vi "cDAQ DDS Open.vi"(8 "error in":errorcluster, 11 "session in":T1={"device"="", "channels"=[], "mclk source"="", "mclk [Hz]"=0.0, "fs [Hz]"=0.0, "block [s]"=0.0, "buf [s]"=0.0, "task"="", "cmd queue"=refnum, "proc ref"=refnum, "smpl clock out"="/cDAQ3/PFI0", "export smpl clock"=FALSE, "DC ofs [V]"=[], "timebase source"="", "timebase mode"=enum."Local"} {"channels" min=0 step=1}) -> (0 "error out":errorcluster, 2 "idn string":string, 3 "session out":T1={"device"="", "channels"=[], "mclk source"="", "mclk [Hz]"=0.0, "fs [Hz]"=0.0, "block [s]"=0.0, "buf [s]"=0.0, "task"="", "cmd queue"=refnum, "proc ref"=refnum, "smpl clock out"="/cDAQ3/PFI0", "export smpl clock"=FALSE, "DC ofs [V]"=[], "timebase source"="", "timebase mode"=enum."Local"} {"channels" min=0 step=1})   [LabVIEW 2020]
uses:
  cDAQ DDS Session.ctl
  cDAQ DDS Setup.ctl
  cDAQ DDS Timebase Mode.ctl
  <vilib>/Utility/error.llb/Error Cluster From Error Code.vi
  <vilib>/DAQmx/create/channels.llb/DAQmx Create Channel (AO-Voltage-Basic).vi
  <vilib>/ErrorRing/Error Ring.xnode
  <resource>/objmgr/daqmx.rc
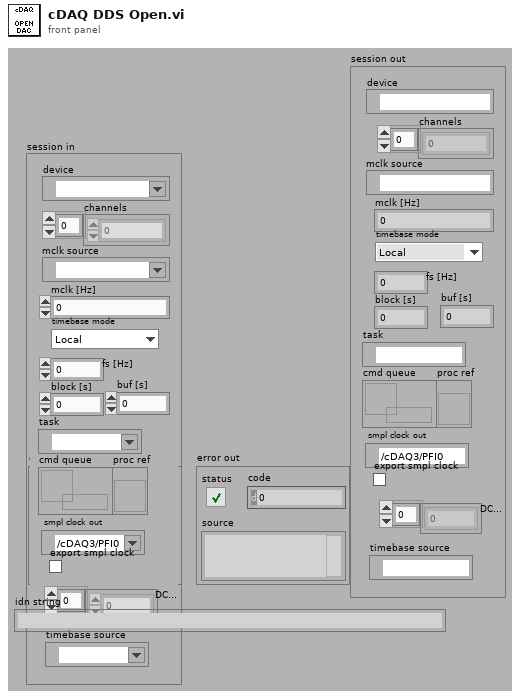
[diagram p1: front panel]
types:
  T1 = typedef "cDAQ DDS Session.ctl" = cluster{"device":tag, "channels":i32[], "mclk source":tag, "mclk [Hz]":dbl, "fs [Hz]":dbl, "block [s]":dbl, "buf [s]":dbl, "task":refnum<k21>, "cmd queue":refnum<queue>, "proc ref":refnum<vi>, "smpl clock out":tag, "export smpl clock":bool, "DC ofs [V]":dbl[], "timebase source":tag, "timebase mode":T2}
  T2 = typedef "cDAQ DDS Timebase Mode.ctl" = enum16{"Local", "Take from ADC (e.g. NI 9238)", "Other source"}
  T3 = typedef "cDAQ DDS Setup.ctl" = cluster{"A [V]":dbl[], "ph [rad]":dbl[], "f [Hz]":dbl[], "stop":bool, "ofs [V]":dbl[]}
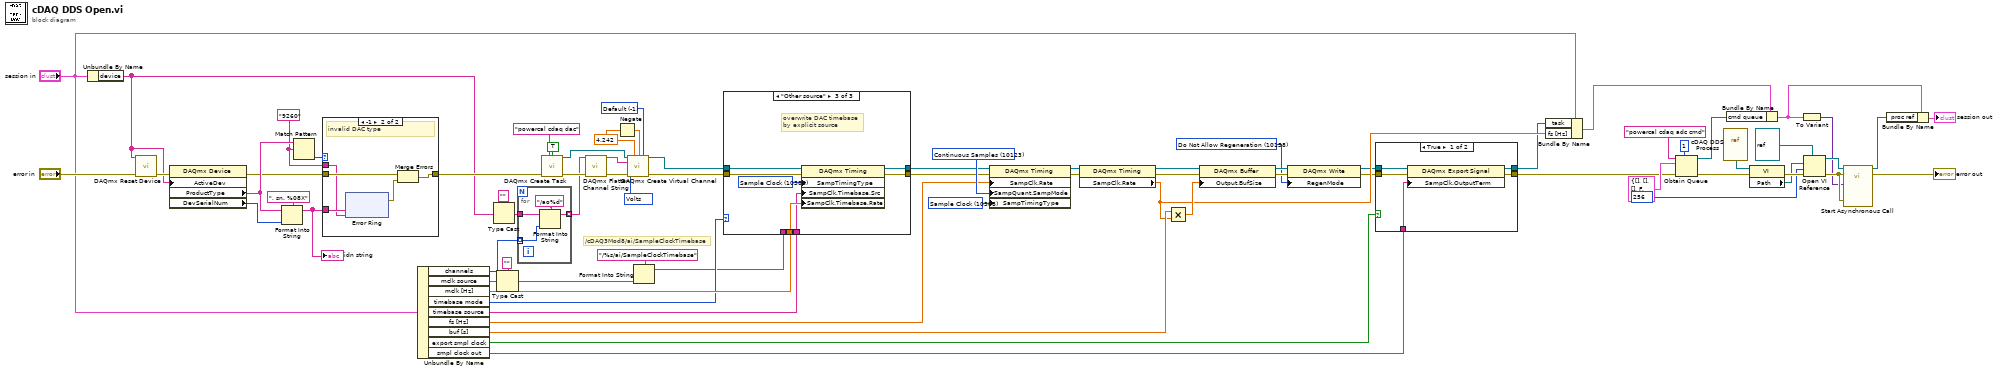
[diagram p0: block diagram]
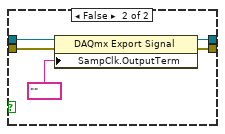
[diagram p2: hidden frame]
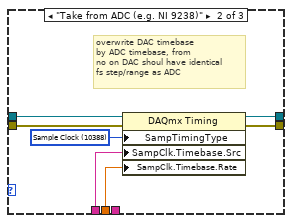
[diagram p4: hidden frame]
diagram:
  w38 = 10158 items=["Allow Regeneration"=10097, "Do Not Allow Regeneration"=10158] ("RegenMode")
  w42 = 10388 items=["Sample Clock"=10388, "Burst Handshake"=12548, "Handshake"=10389, "Implicit"=10451, "On Demand"=10390, "Change Detection"=12504, "Pipelined Sample Clock"=14668] ("SampTimingType")
  w45 = 10123 items=["Finite Samples"=10178, "Continuous Samples"=10123, "Hardware Timed Single Point"=12522] ("SampQuant.SampMode")
  w54 = "9260" ("regular expression")
  w63 = 4.242 ("maximum value")
  w65 = -1 items=["Default"=-1, "RSE"=10083, "Differential"=10106, "Pseudodifferential"=12529] ("output terminal configuration")
  w69 = 10348 items=["Volts"=10348, "From Custom Scale"=10065] ("units")
  # "/cDAQ3Mod8/ai/SampleClockTimebase"
  n1 = Unbundle By Name("session in") -> ("device"=w4:tag)
  n2 = call <vilib>:"DAQmx Reset Device.vi"("device in"=w4, "error in"="error in") -> ("error out"=w61:errorcluster)  [unwired: 13 in]
  n3 = property class="DAQmx Device"(error in=w61, "ActiveDev"=w4) -> (error out=w56:errorcluster, "ProductType"=w58:string, "DevSerialNum"=w60:u32)  [unwired: 1 in, 1 out]
  n4 = Format Into String(format string=", sn. %08X", initial string=w58, w60) -> (resulting string=w55:string)  [unwired: 1 in, 1 out]
  "idn string" <- w55
  n5 = Match Pattern(string=w58, regular expression=w54) -> (offset past match=w57:i32)  [unwired: 1 in, 3 out]
  n6 = case shown="-1" w57 {
    tunnel: w56 -> [w76 w81]
    tunnel: w55 -> [_ w78]
    tunnel: [w76 w79] -> w53
    tunnel: w54 -> [_ w77]
    frame Default {
    }
    frame -1 {
      # "invalid DAC type"
      n7 = xnode "Error Ring"("parameter 0"=w78, "parameter 1"=w77) -> ("error out"=w80:errorcluster)
      n8 = Merge Errors(w81, w80) -> (w79:errorcluster)
    }
  }
  n9 = Unbundle By Name("session in") -> ("channels"=w11:i32[], "mclk source"=w50:tag, "mclk [Hz]"=w47:dbl, "timebase mode"=w3:T2, "timebase source"=w2:tag, "fs [Hz]"=w43:dbl, "buf [s]"=w44:dbl, "export smpl clock"=w6:bool, "smpl clock out"=w5:tag)
  n10 = Type Cast(type="", x=w4) -> (*(type *) &x=w67:string)
  n11 = Type Cast(type="", x=w50) -> (*(type *) &x=w48:string)
  n12 = for {
    tunnel: w67 -> [w92]
    tunnel: [w91] -> w71 mode=indexing
    tunnel: w11 -> [w90] mode=indexing
    n13 = Format Into String(format string="/ao%d", initial string=w92, w90) -> (resulting string=w91:string)  [unwired: 1 in, 1 out]
  }
  n14 = call <vilib>:"DAQmx Create Task.vi"("new task name"="powercal cdaq dac", "auto cleanup"=TRUE, "error in"=w53) -> ("task out"=w74:refnum<k21>, "error out"=w73:errorcluster)  [unwired: 11 in]
  n15 = call <vilib>:"DAQmx Flatten Channel String.vi"("names in"=w71, "error in"=w73) -> ("names out"=w70:string, "error out"=w72:errorcluster)  [unwired: 12 in]
  n16 = Negate(x=w63) -> (-x=w64:dbl)
  n17 = call-poly <vilib>:"DAQmx Create Virtual Channel.vi"("task in"=w74, "maximum value"=w63, "minimum value"=w64, "output terminal configuration"=w65, "physical channels"=w70, "units"=w69, "error in"=w72) -> ("task out"=w46:refnum<k21>, "error out"=w52:errorcluster)  [unwired: 7 in]
  n18 = Format Into String(format string="/%s/ai/SampleClockTimebase", w48) -> (resulting string=w1:string)  [unwired: 2 in, 1 out]
  n19 = case shown="\"Other source\"" w3 {
    tunnel: w52 -> [w95 w101 w108]
    tunnel: w47 -> [_ w100 w107]
    tunnel: w46 -> [w94 w99 w106]
    tunnel: [w95 w98 w105] -> w37
    tunnel: [w94 w97 w104] -> w36
    tunnel: w2 -> [_ _ w103]
    tunnel: w1 -> [_ w96 _]
    frame "Local", Default {
    }
    frame "Take from ADC (e.g. NI 9238)" {
      w102 = 10388 items=["Sample Clock"=10388, "Burst Handshake"=12548, "Handshake"=10389, "Implicit"=10451, "On Demand"=10390, "Change Detection"=12504, "Pipelined Sample Clock"=14668] ("SampTimingType")
      # "overwrite DAC timebase\nby ADC timebase, from\nno on DAC shoul have identical\nfs step/range as ADC"
      n20 = property class="DAQmx Timing"(reference=w99, error in=w101, "SampTimingType"=w102, "SampClk.Timebase.Src"=w96, "SampClk.Timebase.Rate"=w100) -> (reference out=w97:refnum<k21>, error out=w98:errorcluster)
    }
    frame "Other source" {
      w109 = 10388 items=["Sample Clock"=10388, "Burst Handshake"=12548, "Handshake"=10389, "Implicit"=10451, "On Demand"=10390, "Change Detection"=12504, "Pipelined Sample Clock"=14668] ("SampTimingType")
      # "overwrite DAC timebase\nby explicit source"
      n21 = property class="DAQmx Timing"(reference=w106, error in=w108, "SampTimingType"=w109, "SampClk.Timebase.Src"=w103, "SampClk.Timebase.Rate"=w107) -> (reference out=w104:refnum<k21>, error out=w105:errorcluster)
    }
  }
  n22 = property class="DAQmx Timing"(reference=w36, error in=w37, "SampClk.Rate"=w43, "SampQuant.SampMode"=w45, "SampTimingType"=w42) -> (reference out=w34:refnum<k21>, error out=w35:errorcluster)
  n23 = property class="DAQmx Timing"(reference=w34, error in=w35) -> (reference out=w32:refnum<k21>, error out=w33:errorcluster, "SampClk.Rate"=w28:dbl)
  n24 = Multiply(x=w44, y=w28) -> (x*y=w41:dbl)
  n25 = property class="DAQmx Buffer"(reference=w32, error in=w33, "Output.BufSize"=w41) -> (reference out=w39:refnum<k21>, error out=w40:errorcluster)
  n26 = property class="DAQmx Write"(reference=w39, error in=w40, "RegenMode"=w38) -> (reference out=w10:refnum<k21>, error out=w9:errorcluster)
  n27 = case shown="True" w6 {
    tunnel: w10 -> [w114 w119]
    tunnel: w9 -> [w113 w118]
    tunnel: [w112 w117] -> w8
    tunnel: [w111 w116] -> w7
    tunnel: w5 -> [w110 _]
    frame True {
      n28 = property class="DAQmx Export Signal"(reference=w114, error in=w113, "SampClk.OutputTerm"=w110) -> (reference out=w112:refnum<k21>, error out=w111:errorcluster)
    }
    frame False {
      n29 = property class="DAQmx Export Signal"(reference=w119, error in=w118, "SampClk.OutputTerm"=tag "") -> (reference out=w117:refnum<k21>, error out=w116:errorcluster)
    }
  }
  n30 = Bundle By Name(cluster="session in", "task"=w8, "fs [Hz]"=w28) -> (w18:T1)
  n31 = Obtain Queue(max queue size (-1, unlimited)=1, name (unnamed)="powercal cdaq adc cmd", element data type=T3 {"A [V]"=[], "ph [rad]"=[], "f [Hz]"=[], "stop"=FALSE, "ofs [V]"=[]} ("cDAQ dds setup"), error in (no error)=w7) -> (queue out=w16:refnum<queue>, error out=w19:errorcluster)  [unwired: 1 in, 1 out]
  n32 = vi-ref "cDAQ DDS Process.vi"() -> (w26:refnum<vi>)
  n33 = Bundle By Name(cluster=w18, "cmd queue"=w16) -> (w15:T1)
  n34 = property class="VI"(reference=w26, error in=w19) -> (error out=w25:errorcluster, "Path"=w23:path)  [unwired: 1 out]
  n35 = To Variant(anything=w15) -> (Variant=w20:variant)
  n36 = Open VI Reference(type specifier VI Refnum (for type only)=refnum<vi> refnum, vi path=w23, options=256, error in (no error)=w25) -> (vi reference=w27:refnum<vi>, error out=w24:errorcluster)  [unwired: 2 in]
  n37 = call-by-ref "Start Asynchronous Call"(reference=w27, error in=w24, "error in"=w24, "cdaq session"=w20) -> (reference out=w13:refnum<vi>, error out=→"error out":errorcluster)  [unwired: 9 in, 1 out]
  n38 = Bundle By Name(cluster=w15, "proc ref"=w13) -> (→"session out":T1)
